vi "forceconfig.vi"(7 "spc":dbl, 9 "c":dbl, 10 "b":dbl, 11 "a":dbl) -> ()   [LabVIEW 2017, in "HapticSTM.lvlib"]
doc: "extern \"C\" __declspec(dllexport) void forceconfig(double a, double b, double c, double spc);"
uses:
  HapticSTM.lvlib
  <userlib>/HapticSTM/HapticSTM.dll
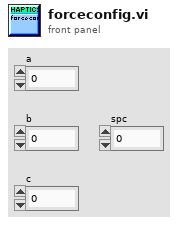
[diagram p1: front panel]
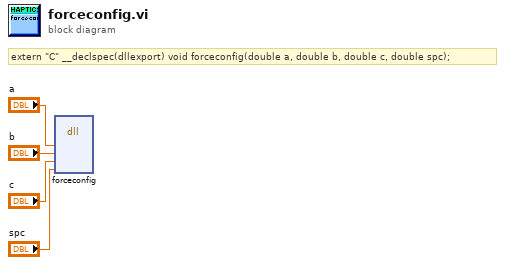
[diagram p0: block diagram]
diagram:
  # "extern \"C\" __declspec(dllexport) void forceconfig(double a, double b, double c, double spc);"
  n1 = dll-call lib="C:/Program Files/National Instruments/LabVIEW 2019/user.lib/HapticSTM/HapticSTM.*" fn="forceconfig"("a"="a", "b"="b", "c"="c", "spc"="spc") -> ()  [unwired: 8 in, 2 out]
